vi "Test MIO Analog Measurement.vi"(7 "Config":T1={"Samples to Read (50)"=50, "Terminal Config (RSE)"=10083, "Channel (0)"=0, "Read Function (Get All)"=enum."Get Latest"} {"Terminal Config (RSE)" items=["Default"=-1, "RSE"=10083, "NRSE"=10078, "Differential"=10106, "Pseudodifferential"=12529]}, 8 "error in (no error)":errorcluster, 9 "Instrument":i32, 10 "Test Label":string, 11 "Test Class in":refnum<class "Test Class.lvclass">) -> (0 "error out":errorcluster, 1 "Result":string, 2 "Passed":bool, 3 "Test Class out":refnum<class "Test Class.lvclass">)   [LabVIEW 2015, in "Test Class.lvclass"]
uses:
  Test Class.lvclass
  Analog MIO Measurement Config -- Cluster.ctl
  Classes/Instruments/MIO Device/Class/typedefs/Read Type -- Enum.ctl
  Classes/Instruments/MIO Device/Class/typedefs/Channel Type -- Enum.ctl
  Classes/Instruments/MIO Device/Class/MIO Device.lvclass
  Test Class.lvclass/Test Class.ctl
  Classes/Application/Class/Application.lvclass
  Classes/Test Recipe/Class/Test Recipe.lvclass
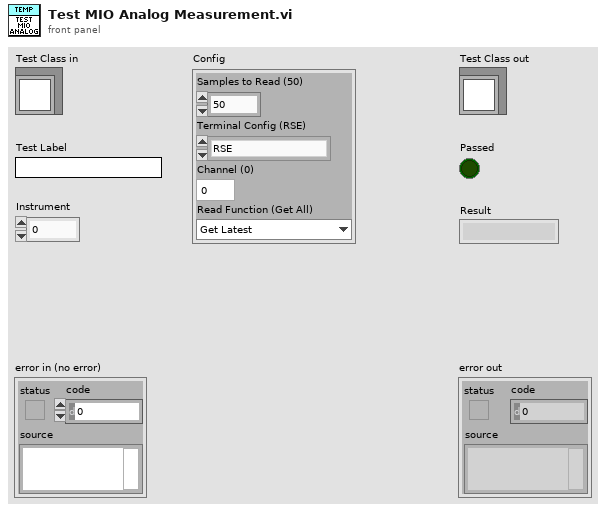
[diagram p1: front panel]
types:
  T1 = typedef "Test Class.lvclass/Analog MIO Measurement Config -- Cluster.ctl" = cluster{"Samples to Read (50)":i32, "Terminal Config (RSE)":i32, "Channel (0)":u32, "Read Function (Get All)":T2}
  T2 = typedef "MIO Device.lvlib/MIO Device.lvclass/Read Type -- Enum.ctl" = enum16{"Get All", "Get Latest", "Get Average"}
  T3 = typedef "MIO Device.lvlib/MIO Device.lvclass/Channel Type -- Enum.ctl" = enum16{"Analog Input", "Analog Output", "Digital Input", "Digital Output"}
  T4 = typedef "Application.lvlib/App Properties.lvclass/Class Properties -- Cluster.ctl" = cluster{"UUT Info":T5[], "Test Information":refnum<vi>, "Test Complete Event":refnum<user-event>, "Shop Floor System":refnum<class "Shop Floor System.lvclass">, "Gold Board":refnum<class "Golden Board.lvclass">, "Test Recipe":refnum<class "Test Recipe.lvclass">, "Instruments":refnum<class "Base Class.lvclass">[], "Mode":T6, "Test Results":cluster{"Pass":bool[], "Fail Codes":string[]}}
  T5 = typedef "Application.lvlib/App Properties.lvclass/UUT Reference -- Cluster.ctl" = cluster{"Serial Number Reference":refnum<vi>, "Status Message Reference":refnum<vi>}
  T6 = typedef "Application.lvlib/Application.lvclass/Op Mode -- Enum.ctl" = u16
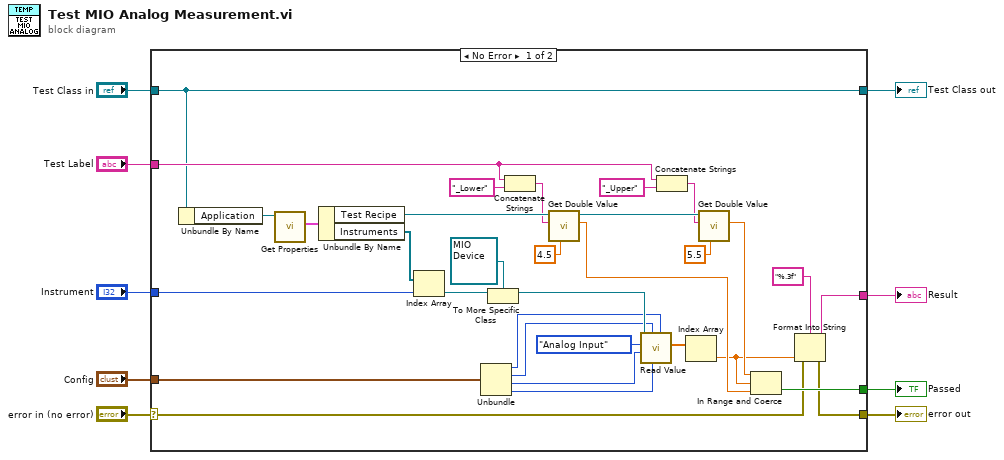
[diagram p0: block diagram]
diagram:
  n1 = case shown="No Error" "error in (no error)" {
    selector: "error in (no error)" -> [w19 w43]
    tunnel: [w18 w43] -> w8
    tunnel: [w17 w42] -> w6
    tunnel: "Test Class in" -> [w17 w42]
    tunnel: "Test Label" -> [w23 _]
    tunnel: [w21 _] -> w4
    tunnel: [w20 _] -> w3
    tunnel: "Instrument" -> [w15 _]
    tunnel: "Config" -> [w14 _]
    frame No Error {
      n2 = Unbundle By Name(w17) -> ("Application"=w16:refnum<class "Application.lvclass">)
      n3 = call "Get Properties.vi"("Acrobat Template in"=w16) -> ("Class Properties"=w39:T4)  [unwired: 8 in, 2 out]
      n4 = Unbundle By Name(w39) -> ("Test Recipe"=w36:refnum<class "Test Recipe.lvclass">, "Instruments"=w40:refnum<class "Base Class.lvclass">[])
      n5 = Index Array(array=w40, index=w15) -> (element=w41:refnum<class "Base Class.lvclass">)
      n6 = Unbundle(w14) -> ("Samples to Read (50)"=w13:i32, "Terminal Config (RSE)"=w12:i32, "Channel (0)"=w11:u32, "Read Function (Get All)"=w10:T2)
      n7 = To More Specific Class(target class=refnum<class "MIO Device.lvclass"> refnum ("MIO Device.lvlib:MIO Device.lvclass"), reference=w41) -> (specific class reference=w38:refnum<class "MIO Device.lvclass">)  [unwired: 1 in, 1 out]
      n8 = Concatenate Strings(w23, "_Lower" ("Name")) -> (w27:string)
      n9 = call "Get Double Value.vi"("Default Value"=4.5, "Name"=w27, "Test Recipe in"=w36) -> ("Value"=w30:dbl, "Test Recipe out"=w35:refnum<class "Test Recipe.lvclass">)  [unwired: 6 in, 1 out]
      n10 = call-dynamic "Read Value.vi"("Samples to Read (50)"=w13, "Read Function (Get All)"=w10, "Terminal Config (RSE)"=w12, "Channel (0)"=w11, "Channel Type"=Channel_Type_--_Enum."Analog Input", "MIO Device in"=w38) -> ("Value"=w32:dbl[])  [unwired: 3 in, 2 out]
      n11 = Concatenate Strings(w23, "_Upper" ("Name")) -> (w25:string)
      n12 = Index Array(array=w32) -> (element=w29:dbl)  [unwired: 1 in]
      n13 = call "Get Double Value.vi"("Default Value"=5.5, "Name"=w25, "Test Recipe in"=w35) -> ("Value"=w31:dbl)  [unwired: 6 in, 2 out]
      n14 = In Range and Coerce(upper limit=w31, x=w29, lower limit=w30) -> (In Range?=w20:bool)  [unwired: 1 out]
      n15 = Format Into String(format string="%.3f", error in=w19, w29) -> (resulting string=w21:string, error out=w18:errorcluster)  [unwired: 1 in]
    }
    frame Error {
    }
  }
  "error out" <- w8
  "Test Class out" <- w6
  "Passed" <- w3
  "Result" <- w4
